vi "Stop Processing.vi"(8 "error in (no error)":errorcluster, 10 "Queue in":refnum<queue>) -> (0 "error out":errorcluster)   [LabVIEW 2023, in "HAF.lvlib" / "TestProcessor.lvclass"]
doc: "All Processing should stop. Send an Exit message to ensure clean shutdown."
uses:
  TestProcessor.lvclass
  TestProcessor.lvclass/TestProcessor.ctl
  HAF.lvlib
  All Internal Message Ids.ctl
  Message.ctl
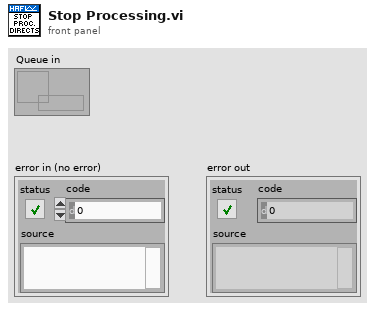
[diagram p1: front panel]
types:
  T1 = typedef "HAF.lvlib/All Internal Message Ids.ctl" = cluster{"Initialise":string, "Process":string, "Continue":string, "Done":string, "Pause":string, "Resume":string, "Stop":string, "Exit":string}
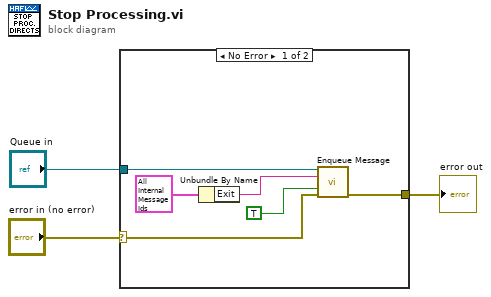
[diagram p0: block diagram]
diagram:
  n1 = case shown="No Error" "error in (no error)" {
    selector: "error in (no error)" -> [w4 w10]
    tunnel: [w9 w10] -> w3
    tunnel: "Queue in" -> [w5 _]
    frame No Error {
      n2 = Unbundle By Name(T1 {"Initialise"="Initialise", "Process"="Process", "Continue"="Continue", "Done"="Done", "Pause"="Pause", "Resume"="Resume", "Stop"="Stop", "Exit"="Exit"} ("Message Ids")) -> ("Exit"=w8:string)
      n3 = call "Enqueue Message.vi"("Message Queue In"=w5, "Message Id"=w8, "Priority"=TRUE, "error in (no error)"=w4) -> ("error out"=w9:errorcluster)  [unwired: 10 in, 1 out]
    }
    frame Error {
    }
  }
  "error out" <- w3
